vi "DataHandler Start.vi"(8 "error in (no error)":errorcluster, 11 "DataProcessor in":refnum<class "DataProcessor.lvclass">) -> (0 "error out":errorcluster, 3 "DataProcessor out":refnum<class "DataProcessor.lvclass">)   [LabVIEW 2020, in "Volatus.lvlib" / "DataProcessor.lvclass"]
uses:
  DataProcessor.lvclass
  C:/Program Files (x86)/National Instruments/LabVIEW 2020/vi.lib/ActorFramework/Actor/Actor.lvclass
  lv-promises/Promises/Promise/Promise.lvclass
  <vilib>/ActorFramework/Actor/Actor.lvclass/Actor.ctl
  <vilib>/ActorFramework/Message Enqueuer/Message Enqueuer.lvclass/Message Enqueuer.ctl
  DataProcessor.lvclass/DataProcessor.ctl
  DataHandler Messages/Register Groups Msg/Register Groups Msg.lvclass/Register Groups Msg.ctl
  <vilib>/ActorFramework/Message Enqueuer/Init from Existing Queue.vi
  <vilib>/ActorFramework/Message Enqueuer/Enqueue.vi
  DataHandler Messages/Register Groups Msg/Register Groups Msg.lvclass
  C:/Program Files (x86)/National Instruments/LabVIEW 2020/vi.lib/ActorFramework/Message/Message.lvclass
  <vilib>/ActorFramework/Message Priority Queue/Priority Enqueue.vi
  <vilib>/ActorFramework/Message Enqueuer/Message Enqueuer.lvclass
  <vilib>/ActorFramework/Actor/Actor.lvclass
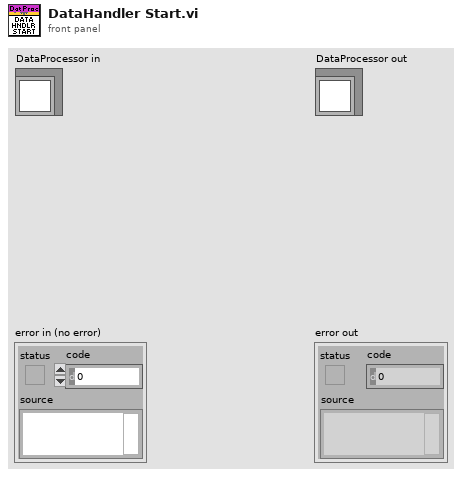
[diagram p1: front panel]
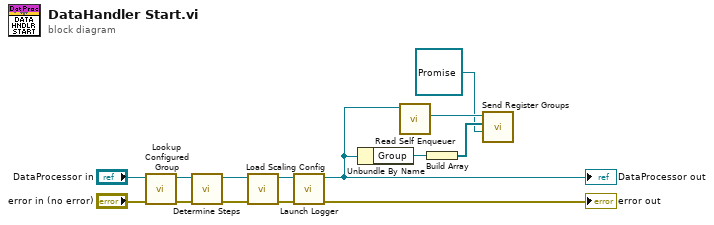
[diagram p0: block diagram]
diagram:
  n1 = call "Lookup Configured Group.vi"("error in (no error)"="error in (no error)", "DataProcessor in"="DataProcessor in") -> ("error out"=w3:errorcluster, "DataProcessor out"=w4:refnum<class "DataProcessor.lvclass">)  [unwired: 8 in]
  n2 = call "Determine Steps.vi"("error in (no error)"=w3, "DataProcessor in"=w4) -> ("error out"=w6:errorcluster, "DataProcessor out"=w5:refnum<class "DataProcessor.lvclass">)  [unwired: 8 in]
  n3 = call "Load Scaling Config.vi"("error in (no error)"=w6, "DataProcessor in"=w5) -> ("error out"=w2:errorcluster, "DataProcessor out"=w1:refnum<class "DataProcessor.lvclass">)  [unwired: 8 in]
  n4 = call "Launch Logger.vi"("error in (no error)"=w2, "DataProcessor in"=w1) -> ("error out"=→"error out":errorcluster, "DataProcessor out"=w8:refnum<class "DataProcessor.lvclass">)  [unwired: 8 in]
  "DataProcessor out" <- w8
  n5 = Unbundle By Name(w8) -> ("Group"=w10:refnum<class "Group.lvclass">)
  n6 = call <vilib>:"Read Self Enqueuer.vi"("Actor"=w8) -> ("Self Enqueuer"=w11:refnum<class "Message Enqueuer.lvclass">)  [unwired: 10 in]
  n7 = Build Array(w10) -> (w9:refnum<class "Group.lvclass">[])
  n8 = call "Send Register Groups.vi"("Promise"=refnum<class "Promise.lvclass"> refnum, "Groups"=w9, "Message Enqueuer"=w11) -> ()  [unwired: 7 in, 2 out]
